vi "test_stopOfNonRunningTaskShouldReturnNoError.vi"(11 "Test Case In":refnum<class "TaskControllerTests.lvclass">) -> (0 "error out":errorcluster, 3 "Test Case Out":refnum<class "TaskControllerTests.lvclass">)   [LabVIEW 2023, in "TaskControllerTests.lvclass"]
uses:
  TaskControllerTests.lvclass
  <vilib>/Astemes/LUnit/Test Case.lvclass/Test Case.ctl
  <vilib>/Astemes/LUnit/Core/LUnit Test Case/Private/Append Pass Result.vi
  <vilib>/Astemes/LUnit/Core/LUnit Test Case/Private/Append Fail Result.vi
  <vilib>/Astemes/LUnit/Core/LUnit Test Case/Private/Run In UI.vi
  <vilib>/Utility/error.llb/Clear Errors.vi
  TLC_Connect/source/LabVIEW/TaskMock/TaskMock.lvclass
  TLC_Connect/source/LabVIEW/TaskController/TaskController.lvclass
  <vilib>/Astemes/LUnit/Test Case.lvclass
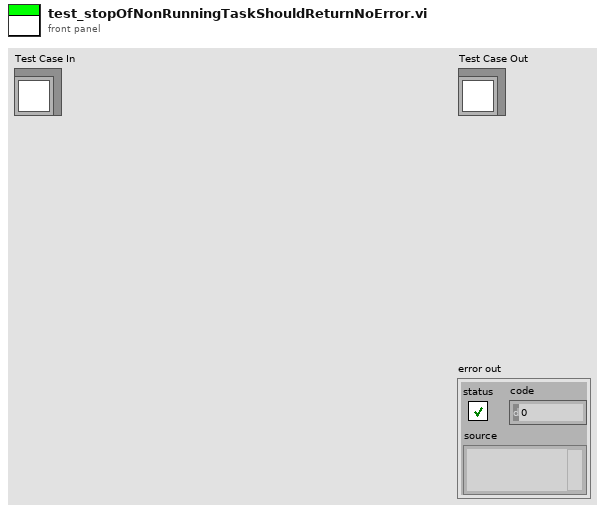
[diagram p1: front panel]
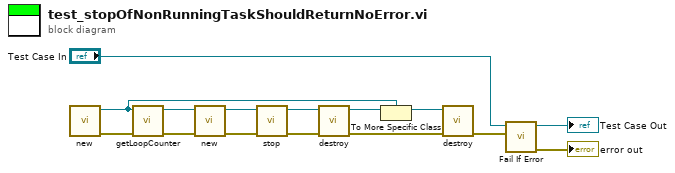
[diagram p0: block diagram]
diagram:
  n1 = call "new.vi"() -> ("error out"=w5:errorcluster, "TaskMock out"=w9:refnum<class "TaskMock.lvclass">)  [unwired: 10 in]
  n2 = call "getLoopCounter.vi"("error in (no error)"=w5, "TaskMock in"=w9) -> ("error out"=w4:errorcluster, "TaskMock out"=w10:refnum<class "TaskMock.lvclass">)  [unwired: 7 in, 1 out]
  n3 = call "new.vi"("error in (no error)"=w4, "task"=w10) -> ("error out"=w11:errorcluster, "TaskController out"=w12:refnum<class "TaskController.lvclass">)  [unwired: 8 in]
  n4 = call "stop.vi"("error in (no error)"=w11, "TaskController in"=w12) -> ("error out"=w3:errorcluster, "TaskController out"=w2:refnum<class "TaskController.lvclass">)  [unwired: 8 in]
  n5 = call "destroy.vi"("error in (no error)"=w3, "TaskController in"=w2) -> ("error out"=w8:errorcluster, "task"=w7:refnum<class "ITask.lvclass">)  [unwired: 8 in]
  n6 = To More Specific Class(target class=w9, reference=w7) -> (specific class reference=w6:refnum<class "TaskMock.lvclass">)  [unwired: 1 in, 1 out]
  n7 = call "destroy.vi"("error in (no error)"=w8, "TaskMock in"=w6) -> ("error out"=w1:errorcluster)  [unwired: 9 in]
  n8 = call <vilib>:"Fail If Error.vi"("Assert error"=w1, "LUnit Test Case In"="Test Case In") -> ("error out"=→"error out":errorcluster, "LUnit Test Case Out"=→"Test Case Out":refnum<class "TaskControllerTests.lvclass">)  [unwired: 8 in]
